vi "MUX Testing.vi"() -> ()   [LabVIEW 2011]
uses:
  <vilib>/ULx/Create Channel.llb/ULx Create Channel (DO-Digital Output).vi
  <vilib>/ULx/Write.llb/ULx Write (Digital U32 1Chan 1Samp).vi
panel:
  in  "Port":refnum<k21>="Dev0/AuxPort"
  # "WATCH THE LEDS!"
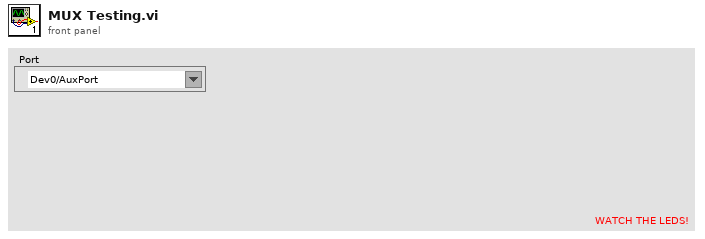
[diagram p1: front panel]
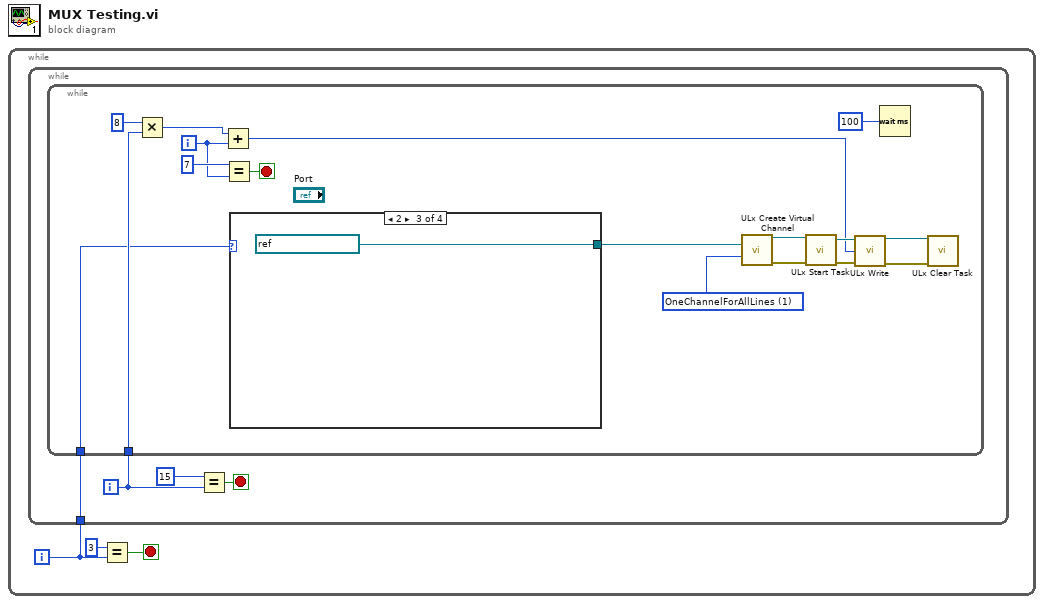
[diagram p0: block diagram]
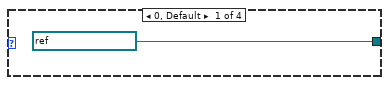
[diagram p2: hidden frame]
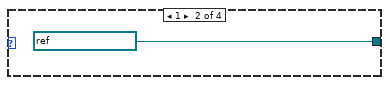
[diagram p3: hidden frame]
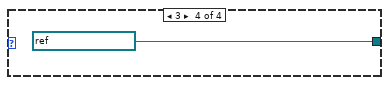
[diagram p4: hidden frame]
diagram:
  n1 = while {
    i -> [w1]
    stop <- w2 stop-if-true
    n2 = while {
      tunnel: w1 -> [w4]
      i -> [w7]
      stop <- w5 stop-if-true
      n3 = while {
        tunnel: w7 -> [w10]
        tunnel: w4 -> [w9]
        i -> [w12]
        stop <- w11 stop-if-true
        w23 = 1 items=["OneChannelForEachLine", "OneChannelForAllLines"] ("line grouping")
        n4 = Multiply(x=8, y=w10) -> (x*y=w15:i32)
        n5 = Add(x=w15, y=w12) -> (x+y=w14:i32)
        n6 = Equal?(x=7, y=w12) -> (x = y?=w11:bool)
        n7 = case shown="2" w9 {
          tunnel: [refnum<k21> "Dev0/1stPortA" ("Port 2") refnum<k21> "Dev0/1stPortB" ("Port 2") refnum<k21> "Dev1/1stPortA" ("Port 2") refnum<k21> "Dev1/1stPortB" ("Port 2")] -> w24
          frame 0, Default {
          }
          frame 1 {
          }
          frame 2 {
          }
          frame 3 {
          }
        }
        n8 = call-poly <vilib>:"ULx Create Virtual Channel.vi"("lines"=w24, "line grouping"=w23) -> ("task out"=w21:refnum<k24>, "error out"=w22:errorcluster)  [unwired: 12 in]
        n9 = call <vilib>:"ULx Start Task.vi"("task in"=w21, "error in"=w22) -> ("task out"=w18:refnum<k24>, "error out"=w17:errorcluster)  [unwired: 12 in]
        n10 = call-poly <vilib>:"ULx Write.vi"("task in"=w18, "data"=w14, "error in"=w17) -> ("task out"=w20:refnum<k24>, "error out"=w19:errorcluster)  [unwired: 10 in, 1 out]
        n11 = Wait (ms)(milliseconds to wait=100) -> ()  [unwired: 1 out]
        n12 = call <vilib>:"ULx Clear Task.vi"("task in"=w20, "error in"=w19) -> ()  [unwired: 13 in, 1 out]
      }
      n13 = Equal?(x=15, y=w7) -> (x = y?=w5:bool)
    }
    n14 = Equal?(x=3, y=w1) -> (x = y?=w2:bool)
  }
